vi "Custom or Standard Message.vi"(0 "Custom Message":string, 1 "Standard Message":string) -> (2 "Message":string)   [LabVIEW 2013, in "Caraya.lvlib"]
uses:
  Caraya.lvlib
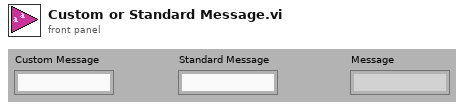
[diagram p1: front panel]
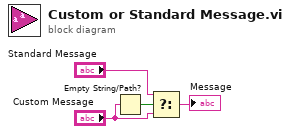
[diagram p0: block diagram]
diagram:
  n1 = Empty String/Path?(string/path="Custom Message") -> (empty?=w4:bool)
  n2 = Select(t="Standard Message", s=w4, f="Custom Message") -> (s? t:f=→"Message":string)
